vi "SpectrumCalibrate.vi"(8 "error in (no error)":errorcluster, 10 "Graph In":refnum<vi>, 11 "Instruments in":refnum<class "Instruments.lvclass">) -> (0 "error out":errorcluster, 1 "max value":dbl, 2 "Integration Time":i32, 3 "Instruments out":refnum<class "Instruments.lvclass">, 4 "Saturated?":bool, 5 "In Range?":bool)   [LabVIEW 2012, in "Instruments.lvclass"]
uses:
  Instruments.lvclass
  Controls/SpectrometerOphirSelector.ctl
  Instruments.lvclass/Instruments.ctl
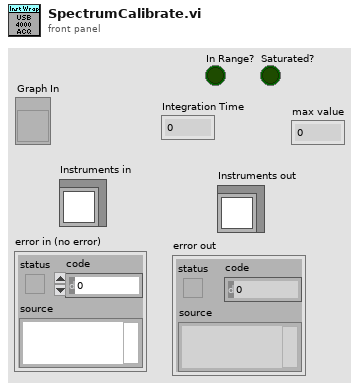
[diagram p1: front panel]
types:
  T1 = typedef "SpectrometerOphirSelector.ctl" = enum16{"Get Background", "Measure", "Measure50", "Raw"}
  T2 = typedef "USB4000_Data.ctl" = cluster{"Wrapper Out":u32, "Number of Spectrometers":i32, "Wavelength":dbl[], "EL Spectrum":dbl[], "Int Time (usec)":i32, bool, "Background":dbl[]}
  T3 = cluster{"Wavelength":dbl[], "EL Spectrum":dbl[]}[]
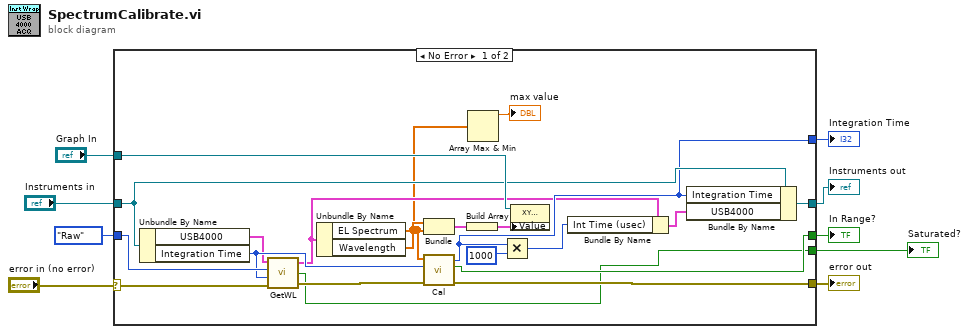
[diagram p0: block diagram]
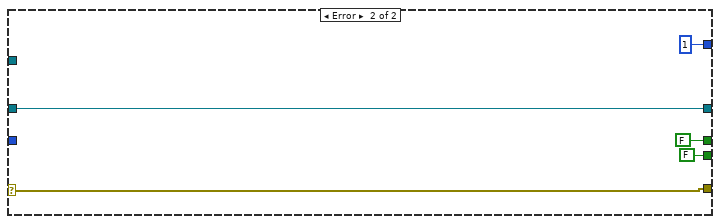
[diagram p2: hidden frame]
diagram:
  n1 = case shown="No Error" "error in (no error)" {
    selector: "error in (no error)" -> [w28 w35]
    tunnel: [w26 w35] -> w8
    tunnel: [w22 w34] -> w6
    tunnel: "Instruments in" -> [w24 w34]
    tunnel: SpectrometerOphirSelector."Raw" ("Type") -> [w30 _]
    tunnel: "Graph In" -> [w25 _]
    tunnel: [w21 1 ("Integration Time")] -> w3
    tunnel: [w13 FALSE ("In Range?")] -> w2
    tunnel: [w12 FALSE ("Saturated?")] -> w1
    frame No Error {
      n2 = Unbundle By Name(w24) -> ("USB4000"=w27:T2, "Integration Time"=w29:i32)
      n3 = call "GetWL.vi"("error in (no error)"=w28, "Integration Time"=w29, "Type"=w30, "USB4000 Params In"=w27) -> ("error out"=w20:errorcluster, "Saturated?"=w12:bool, "USB4000 Params Out"=w16:T2)
      n4 = Unbundle By Name(w16) -> ("EL Spectrum"=w11:dbl[], "Wavelength"=w19:dbl[])
      n5 = Bundle("Wavelength"=w19, "EL Spectrum"=w11) -> (w18:cluster{"Wavelength":dbl[], "EL Spectrum":dbl[]})  [unwired: 1 in]
      n6 = call "Cal.vi"("error in (no error)"=w20, "Int Time(ms)"=w29, "Spectrum"=w11) -> ("error out"=w26:errorcluster, "In Range?"=w13:bool, "NewInt"=w21:i32)  [unwired: 6 in]
      n7 = Build Array(w18) -> (w17:T3)
      n8 = Array Max & Min(array=w11) -> (max value=→"max value":dbl)  [unwired: 3 out]
      n9 = Multiply(x=w21, y=1000 ("NewInt")) -> (x*y=w14:i32)
      n10 = property class="XYGraph (strict)"(reference=w25, "Value"=w17) -> ()  [unwired: 1 in, 2 out]
      n11 = Bundle By Name(cluster=w16, "Int Time (usec)"=w14) -> (w23:T2)
      n12 = Bundle By Name(cluster=w24, "Integration Time"=w21, "USB4000"=w23) -> (w22:refnum<class "Instruments.lvclass">)
    }
    frame Error {
    }
  }
  "error out" <- w8
  "Instruments out" <- w6
  "Integration Time" <- w3
  "In Range?" <- w2
  "Saturated?" <- w1
